vi "PoseStrikerPass.vi"(4 "Field defense":dbl[](array[numeric]), 6 "Array":dbl[](array[numeric]), 7 "AI Parameters":T5={"GotoKick"={"Dist do cone a frente"=150.0, "attacker farback"=1500.0, "Perto"=300.0, "min dist to kick"=150.0, "kick eps"=0.0, "Time to transition"=0.05}, "Attacker"={"CC chute"=0.09, "CC passe"=0.045, "Kick Force"=100.0, "D ball-robot Kick"=200.0, "D ball-robot Pass"=0.3}, "Defender"={"D max"=1700.0, "Vel p/ robô av"=1000.0, "Kick Force"=100.0, "D atk-def"=0.0, "D farback"=0.0}, "Timeout"={"Field/v in x"=6.0, "Dist Robots"=300, "Dist up in y"=300}, "Pose Striker"={"dist"=200.0, "Numeric"=-4.0, "dist 2"=200.0}, "Dist Stop"=300.0, "Distance when ball out"=200, "D central gap "=150.0, "T pass"=0.0, "Force ++"=0.0, "range kick"=0.0, "Chute alto"=TRUE, "Marcador novo"=TRUE} {"D central gap" format="%#_13g"; "Dist Stop" format="%#_13g"; "Pose Striker"."Numeric" format="%#_13g"; "Defender"."Kick Force" format="%#_13g"; "Defender"."Vel p/ robô av" format="%#_13g"; "Attacker"."D ball-robot Kick" format="%#_13g"; "Attacker"."Kick Force" format="%#_13g"; "Attacker"."CC passe" format="%#_13g"; "Attacker"."CC chute" format="%#_13g"; "GotoKick"."kick eps" format="%#_13g"; "GotoKick"."min dist to kick" format="%#_13g"; "GotoKick"."Perto" format="%#_13g"; "GotoKick"."attacker farback" format="%#_13g"; "GotoKick"."Dist do cone a frente" format="%#_13g"}, 8 "atacando ao contrário?":bool=TRUE, 9 "balls":T4[](array[typedef])=[{"x"=-2165.869384765625, "y"=510.4085693359375, "timestamp"=timestamp(2082758857.4639893 s since 1904-01-01), "Vel_x"=0.0, "Vel_y"=0.0, "Pos Bola Est"=[]}], 10 "Robot in":T1={"id"=5, "function"=enum."Attacker", "x"=-1842.5054931640625, "y"=520.60986328125, "orientation"=-2.7555055618286133, "v_tangent"=0.0, "v_normal"=0.0, "v_ang"=0.0, "kick_x"=0.0, "kick_z"=0.0, "dribble"=FALSE, "Timestamp"=timestamp(2082758857.4639893 s since 1904-01-01), "dest_x"=0.0, "dest_y"=0.0, "dest_orientation"=0.0, "estimatives"={"est_v_tangent"=0.0, "est_v_normal"=0.0, "est_vx"=0.0, "est_vy"=0.0, "Pos Robot Est"=[]}, "dest_x_kick"=0.0, "dest_y_kick"=0.0, "Gap Coord"=[], "States"=enum."GoToTangent"}, 11 "IA Input":T6={"our_robots"=[], "enemy_robots"=[], "balls"=[], "geometry"={"line_width"=0, "field_length"=0, "field_width"=0, "boundary_width"=0, "referee_width"=0, "goal_width"=0, "goal_depth"=0, "goal_wall_width"=0, "center_circle_radius"=0, "defense_radius"=0, "defense_stretch"=0, "free_kick_from_defense_dist"=0, "penalty_spot_from_field_line_dist"=0, "penalty_line_from_spot_dist"=0}, "IA Judge"={"stage"="", "command"="", "our_goalie_id"=0.0, "enemy_goalie_id"=0.0, "command enum"=enum."Halt", "Time"=enum."Azul"}, "Received Timestamp"=timestamp(0 s since 1904-01-01), "Events"={"Touch"=FALSE, "Ball out"=FALSE, "id touch"=0.0, "Ball out of \nVision"=FALSE, "Ball inside \nGoalie area"=FALSE, "Robot not responding"=FALSE, "Robots responding status"=[1.0, 1.0, 1.0, 1.0, 1.0, 1.0], "Enemy Ball \nPossession"=FALSE, "Pass State"=FALSE, "id end of pass"=0.0, "Kick"=FALSE, "Id ini Possession"=0.0, "Ball Possesion"=FALSE, "Id Possesion"=0.0}}) -> (2 "Robot out":T1={"id"=5, "function"=enum."Attacker", "x"=-1842.5054931640625, "y"=520.60986328125, "orientation"=-2.7555055618286133, "v_tangent"=-0.08361641967936218, "v_normal"=-0.20513016702014014, "v_ang"=0.24456003022714357, "kick_x"=0.0, "kick_z"=0.0, "dribble"=FALSE, "Timestamp"=timestamp(2082758857.4639893 s since 1904-01-01), "dest_x"=0.0, "dest_y"=0.0, "dest_orientation"=0.0, "estimatives"={"est_v_tangent"=0.0, "est_v_normal"=0.0, "est_vx"=0.0, "est_vy"=0.0, "Pos Robot Est"=[]}, "dest_x_kick"=0.0, "dest_y_kick"=0.0, "Gap Coord"=[], "States"=enum."GoToTangent"})   [LabVIEW 2017]
uses:
  Core/AI Input.ctl
  Core/AI Robot.ctl
  Functions Enum.ctl
  AttackerStates.ctl
  Core/AI Ball.ctl
  Core/Field Size.ctl
  Core/AI Judge.ctl
  Command Enum.ctl
  Util/Events/Events.ctl
  AI Parameters.ctl
panel:
  in  "Time Target (s)":dbl=1.0 format="%#_13g"
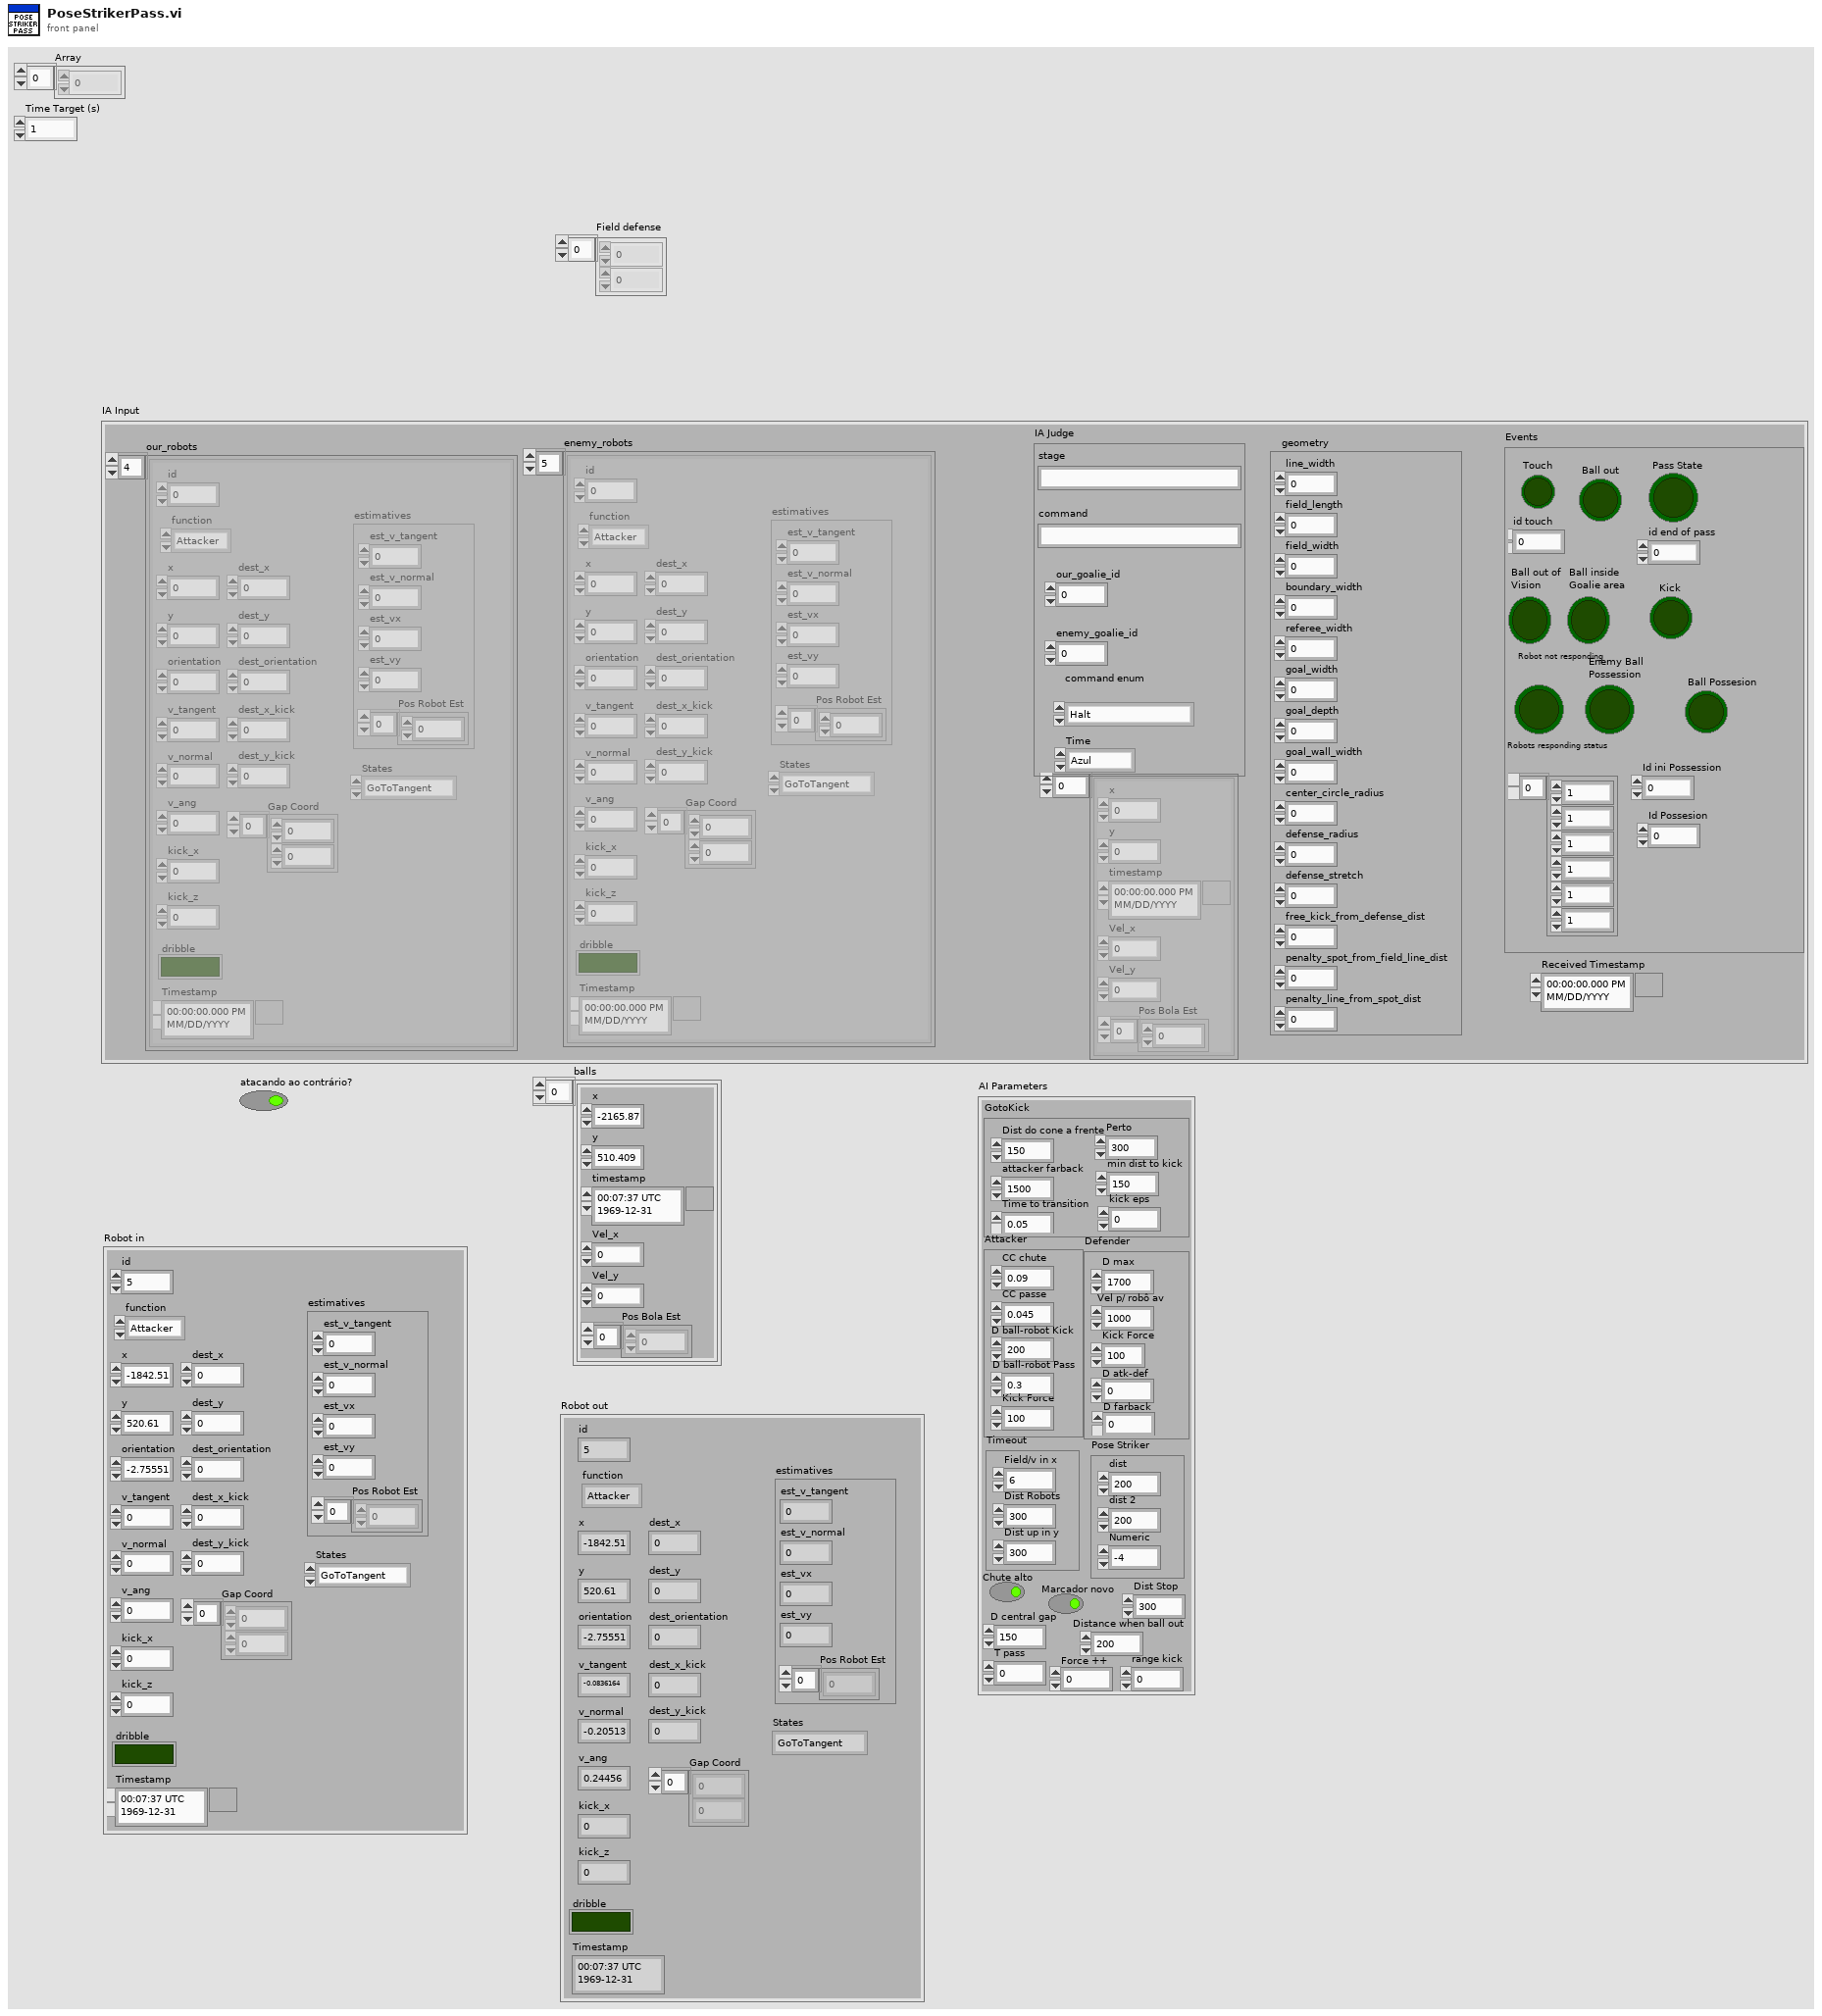
[diagram p1: front panel]
types:
  T1 = typedef "AI Robot.ctl" = cluster{"id":u32, "function":T2, "x":dbl, "y":dbl, "orientation":dbl, "v_tangent":dbl, "v_normal":dbl, "v_ang":dbl, "kick_x":dbl, "kick_z":dbl, "dribble":bool, "Timestamp":timestamp, "dest_x":dbl, "dest_y":dbl, "dest_orientation":dbl, "estimatives":cluster{"est_v_tangent":dbl, "est_v_normal":dbl, "est_vx":dbl, "est_vy":dbl, "Pos Robot Est":dbl[]}, "dest_x_kick":dbl, "dest_y_kick":dbl, "Gap Coord":dbl[], "States":T3}
  T2 = typedef "Functions Enum.ctl" = enum16{"Attacker", "Goalie", "Defender", "Striker", "Goto 0", "Dummy", "Kicker", "ZigZag"}
  T3 = typedef "AttackerStates.ctl" = enum16{"Pass", "GoToTangent", "BallGetting", "GoToKick", ""}
  T4 = typedef "AI Ball.ctl" = cluster{"x":dbl, "y":dbl, "timestamp":timestamp, "Vel_x":dbl, "Vel_y":dbl, "Pos Bola Est":dbl[]}
  T5 = typedef "AI Parameters.ctl" = cluster{"GotoKick":cluster{"Dist do cone a frente":dbl, "attacker farback":dbl, "Perto":dbl, "min dist to kick":dbl, "kick eps":dbl, "Time to transition":dbl}, "Attacker":cluster{"CC chute":dbl, "CC passe":dbl, "Kick Force":dbl, "D ball-robot Kick":dbl, "D ball-robot Pass":dbl}, "Defender":cluster{"D max":dbl, "Vel p/ robô av":dbl, "Kick Force":dbl, "D atk-def":dbl, "D farback":dbl}, "Timeout":cluster{"Field/v in x":dbl, "Dist Robots":u32, "Dist up in y":u32}, "Pose Striker":cluster{"dist":dbl, "Numeric":dbl, "dist 2":dbl}, "Dist Stop":dbl, "Distance when ball out":i32, "D central gap ":dbl, "T pass":dbl, "Force ++":dbl, "range kick":dbl, "Chute alto":bool, "Marcador novo":bool}
  T6 = typedef "AI Input.ctl" = cluster{"our_robots":T1[], "enemy_robots":T1[], "balls":T4[], "geometry":T7, "IA Judge":T8, "Received Timestamp":timestamp, "Events":T10}
  T7 = typedef "Field Size.ctl" = cluster{"line_width":u32, "field_length":u32, "field_width":u32, "boundary_width":u32, "referee_width":u32, "goal_width":u32, "goal_depth":u32, "goal_wall_width":u32, "center_circle_radius":u32, "defense_radius":u32, "defense_stretch":u32, "free_kick_from_defense_dist":u32, "penalty_spot_from_field_line_dist":u32, "penalty_line_from_spot_dist":u32}
  T8 = typedef "AI Judge.ctl" = cluster{"stage":string, "command":string, "our_goalie_id":dbl, "enemy_goalie_id":dbl, "command enum":T9, "Time":enum16{"Azul", "Amarelo"}}
  T9 = typedef "Command Enum.ctl" = enum16{"Halt", "Stop", "Force Start", "PKA Normal Start", "Prepare Kickoff Ally", "PKE Normal Start", "Prepare Kickoff Enemy", "Prepare Penalty Ally", "PPA Normal Start", "Prepare Penalty Enemy", "PPE Normal Start", "Direct Free Enemy", "Direct Free Ally", "Indirect Free Enemy", "Indirect Free Ally", "Timeout Enemy", "Timeout Ally", "Goal Enemy", "Goal Ally", "Ball Placement Enemy", "Ball Placement Ally", "Normal Half Time", "Extra Time Break", "Extra Half Time", "None", "Post Game"}
  T10 = typedef "Events.ctl" = cluster{"Touch":bool, "Ball out":bool, "id touch":dbl, "Ball out of \nVision":bool, "Ball inside \nGoalie area":bool, "Robot not responding":bool, "Robots responding status":dbl[], "Enemy Ball \nPossession":bool, "Pass State":bool, "id end of pass":dbl, "Kick":bool, "Id ini Possession":dbl, "Ball Possesion":bool, "Id Possesion":dbl}
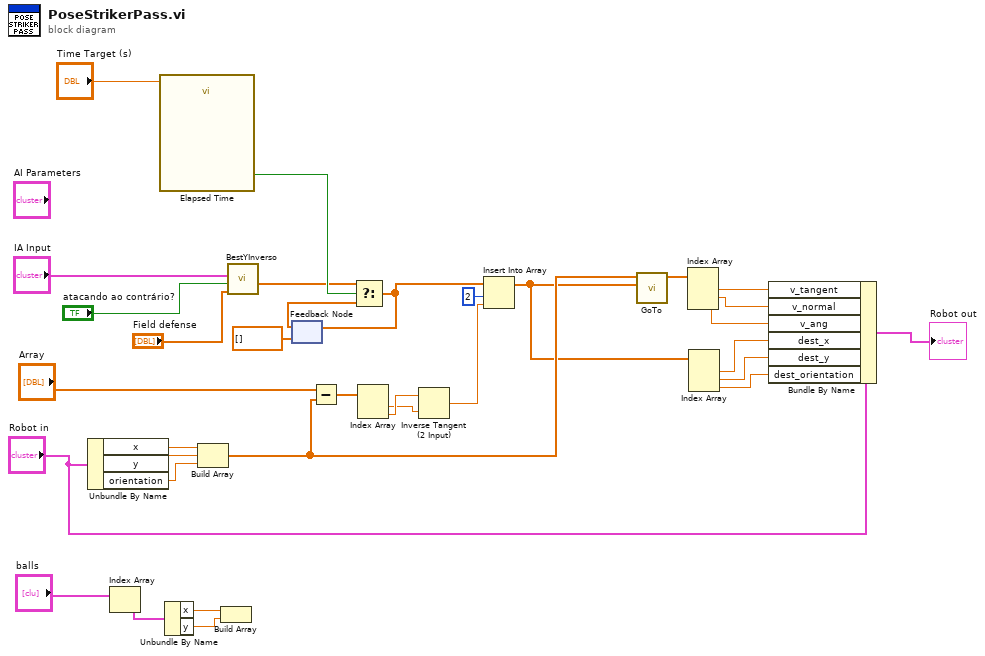
[diagram p0: block diagram]
diagram:
  n1 = Unbundle By Name("Robot in") -> ("x"=w29:dbl, "y"=w28:dbl, "orientation"=w9:dbl)
  n2 = Index Array(array="balls") -> (element=w30:T4)  [unwired: 1 in]
  n3 = call "Elapsed Time"("Time Target (s)"="Time Target (s)") -> ("Time has Elapsed"=w6:bool)  [unwired: 11 in, 7 out]
  n4 = Unbundle By Name(w30) -> ("x"=w27:dbl, "y"=w26:dbl)
  n5 = Build Array(w29, w28, w9) -> (w20:dbl[])
  n6 = Build Array(w27, w26) -> ()  [unwired: 1 out]
  n7 = call "BestYInverso.vi"("Field defense"="Field defense", "atacando contra"="atacando ao contrário?", "IA State"="IA Input") -> ("Position"=w5:dbl[])  [unwired: 8 in]
  n8 = feedback #1(dbl[] [] ("Position")) -> (w4:dbl[])
  n9 = Subtract(x="Array", y=w20) -> (x-y=w25:dbl[])
  n10 = Select(t=w5, s=w6, f=w4) -> (s? t:f=w2:dbl[])
  n11 = feedback-in #1(w2) -> ()
  n12 = Index Array(array=w25) -> (element #1=w23:dbl, element #2=w24:dbl)  [unwired: 2 in]
  n13 = Inverse Tangent (2 Input)(1:w23, 2:w24) -> (0:w22:dbl)
  n14 = Insert Into Array(array=w2, index=2, new element=w22) -> (w15:dbl[])
  n15 = call "GoTo.vi"("Target"=w15, "Position"=w20) -> ("Output\nVelocity"=w19:dbl[])  [unwired: 8 in, 1 out]
  n16 = Index Array(array=w19) -> (element #1=w18:dbl, element #2=w17:dbl, element #3=w16:dbl)  [unwired: 3 in]
  n17 = Index Array(array=w15) -> (element #1=w14:dbl, element #2=w13:dbl, element #3=w12:dbl)  [unwired: 3 in]
  n18 = Bundle By Name(cluster="Robot in", "v_tangent"=w18, "v_normal"=w17, "v_ang"=w16, "dest_x"=w14, "dest_y"=w13, "dest_orientation"=w12) -> (→"Robot out":T1)
